vi "WriteRasterProperties.vi"(4 "Direction Tx0":T1, 6 "Polarization, V0 H1":T2, 8 "error in (no error)":errorcluster, 9 "Window, cm":dbl=42.0, 10 "Nyquist, mm":dbl=28.0, 11 "aparCfg in":refnum<class "aparCfg.lvclass">) -> (0 "error out":errorcluster, 3 "aparCfg out":refnum<class "aparCfg.lvclass">)   [LabVIEW 2017]
uses:
  aparCfg.lvclass
  Sequence/SequenceSubvis/PolarizationSelect.ctl
  Sequence/SequenceSubvis/RF Direction.ctl
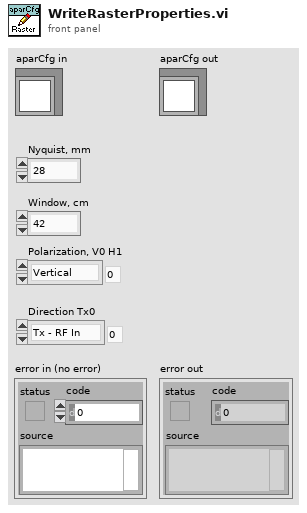
[diagram p1: front panel]
types:
  T1 = typedef "RF Direction.ctl" = enum16{"Tx - RF In", "Rx - RF Out"}
  T2 = typedef "PolarizationSelect.ctl" = enum16{"Vertical", "Horizontal"}
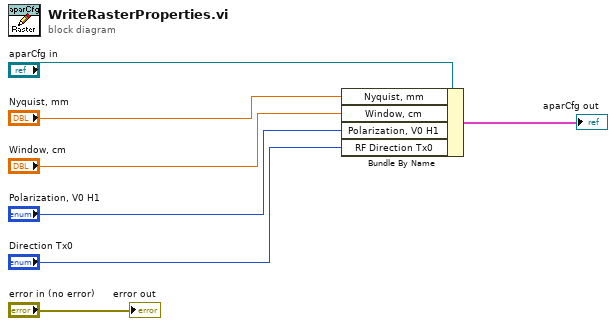
[diagram p0: block diagram]
diagram:
  n1 = Bundle By Name(cluster="aparCfg in", "Nyquist, mm"="Nyquist, mm", "Window, cm"="Window, cm", "Polarization, V0 H1"="Polarization, V0 H1", "RF Direction Tx0"="Direction Tx0") -> (→"aparCfg out":cluster{})
  "error out" <- "error in (no error)"
